vi "Taiko_SimpleDemo.vi"() -> ()   [LabVIEW 2017]
uses:
  _lib/PDLM/pdlm_lib_x86_x64_UIThread.llb/PDLM_LHData.ctl
  _lib/PDLM/pdlm_lib_x86_x64_UIThread.llb/PDLM_LHData_LaserType.ctl
  _lib/PDLM/pdlm_lib_x86_x64_UIThread.llb/PDLM_LHVersion.ctl
  _lib/PDLM/pdlm_lib_x86_x64_UIThread.llb/PDLM_SystemStatus.ctl
  _lib/PDLM/pdlm_lib_x86_x64_UIThread.llb/PDLM_LaserMode.ctl
  _lib/PDLM/pdlm_lib_x86_x64_UIThread.llb/PDLM_TaggedValueList.ctl
  _lib/PDLM/pdlm_lib_x86_x64_UIThread.llb/PDLM_TaggedValue.ctl
  _lib/PDLM/pdlm_lib_x86_x64_UIThread.llb/PDLM_Tag.ctl
  <vilib>/Utility/error.llb/Error Cluster From Error Code.vi
  _lib/PDLM/pdlm_lib_x86_x64_UIThread.llb/PDLM_DllPath_global.vi
  <vilib>/ErrorRing/Error Ring.xnode
panel:
  out "Errror":errorcluster
  in  "Exit":bool
  in  "Update":bool
  out "String":string
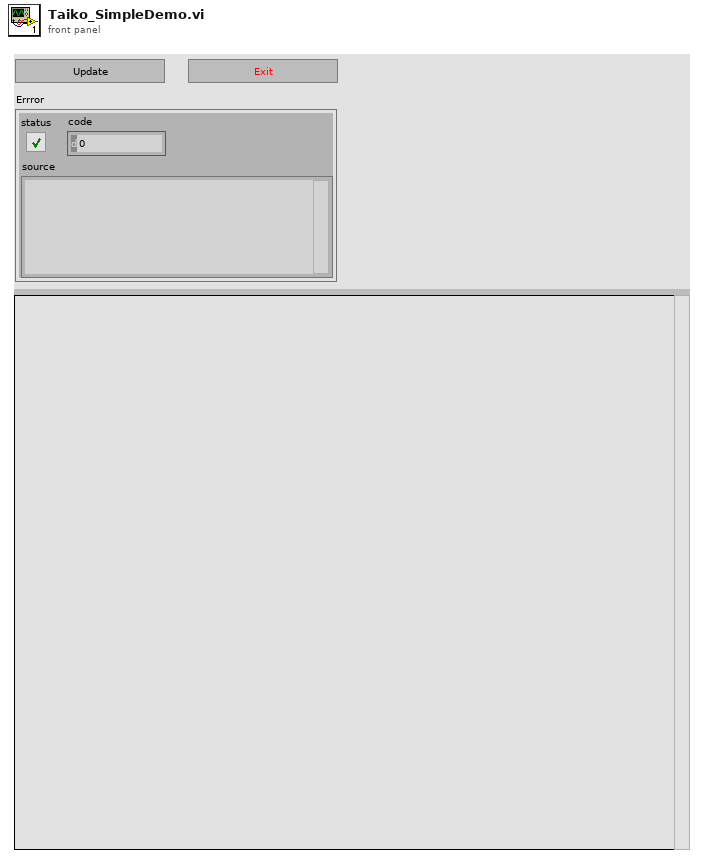
[diagram p1: front panel]
types:
  T1 = typedef "PDLM_LHData.ctl" = cluster{"SerNo":u32, "Features":u32, "FreqMin":u32, "FreqMax":u32, "CwPowerMax":u32, "PulsePowerMax":u32, "WavelengthNominal":u16, "CaseTempMax":u16, "Protection":bool, "LHTypeCtrlVoltage":u16, "LHMaxVoltage":u16, "CurrentTEP12V":u16, "LaserType":T2, "LHVersion":T3, "CalWarrentHours":u16}
  T2 = typedef "PDLM_LHData_LaserType.ctl" = u16
  T3 = typedef "PDLM_LHVersion.ctl" = cluster{"Major":u16, "Minor":u16}
  T4 = typedef "PDLM_LaserMode.ctl" = enum32{"CW", "PULSE", "BURST"}
  T5 = typedef "PDLM_TaggedValueList.ctl" = T6[]
  T6 = typedef "PDLM_TaggedValue.ctl" = cluster{"Tag":T7, "Value":u32}
  T7 = typedef "PDLM_Tag.ctl" = u32
  T8 = typedef "PDLM_SystemStatus.ctl" = u32
  T9 = typedef "PDLM_LHInfo.ctl" = cluster{"LType":string, "Date":string, "LClass":string}
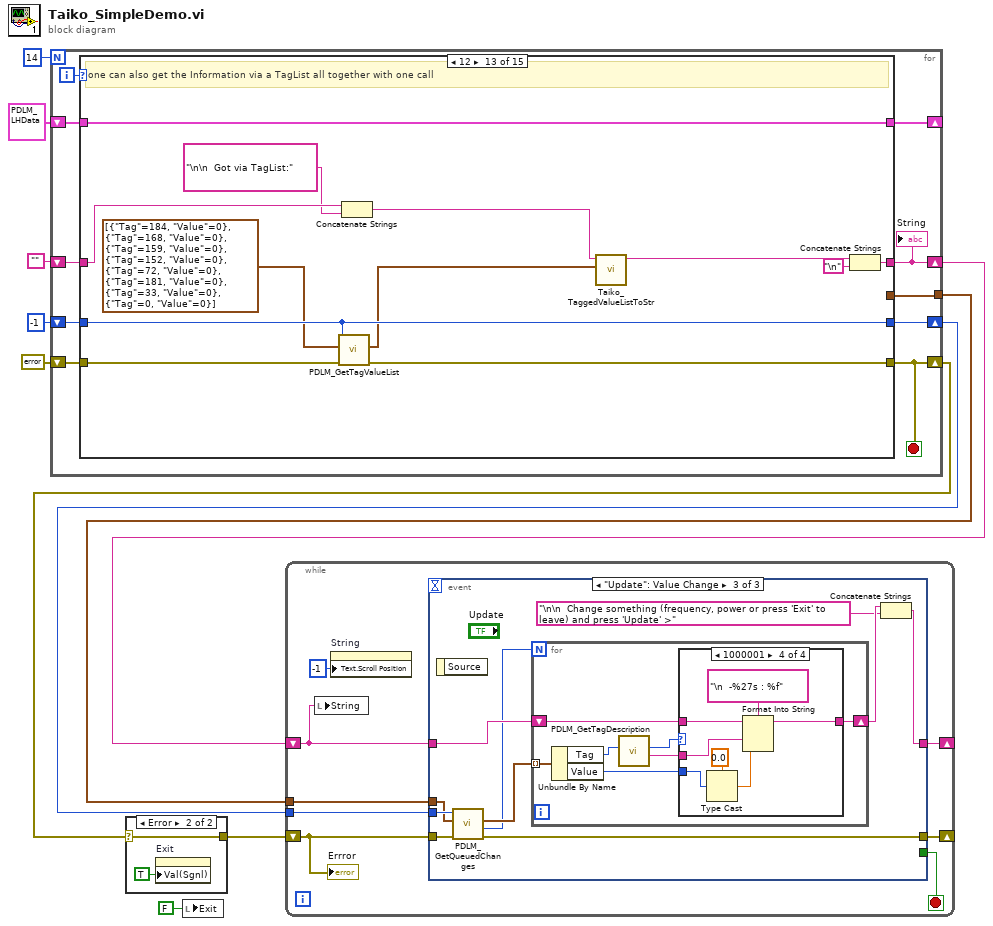
[diagram p0: block diagram]
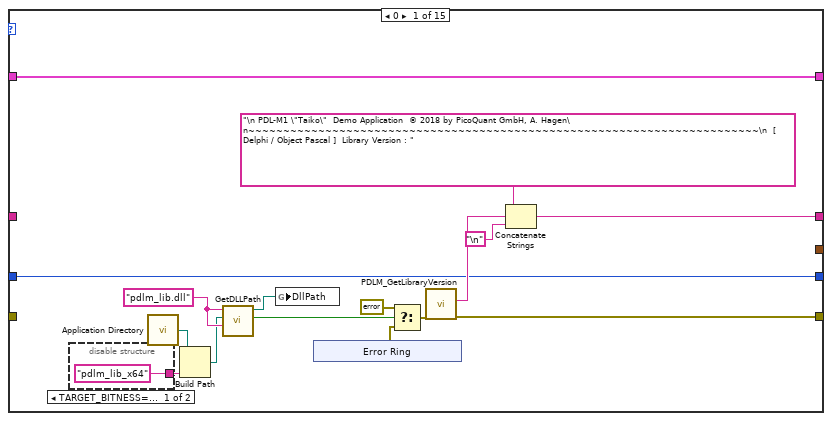
[diagram p3: hidden frame]
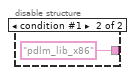
[diagram p4: hidden frame]
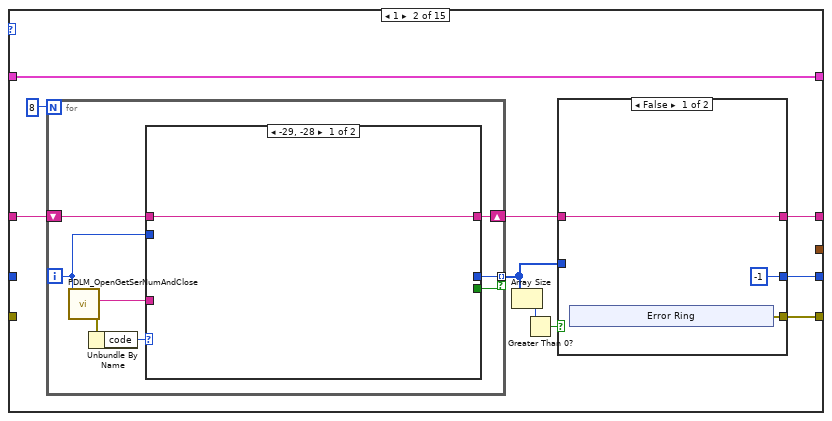
[diagram p5: hidden frame]
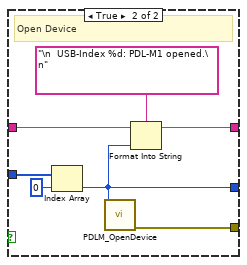
[diagram p6: hidden frame]
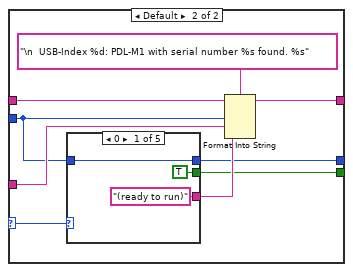
[diagram p7: hidden frame]
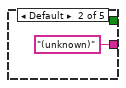
[diagram p8: hidden frame]
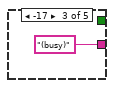
[diagram p9: hidden frame]
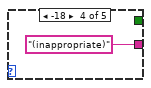
[diagram p10: hidden frame]
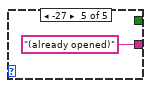
[diagram p11: hidden frame]
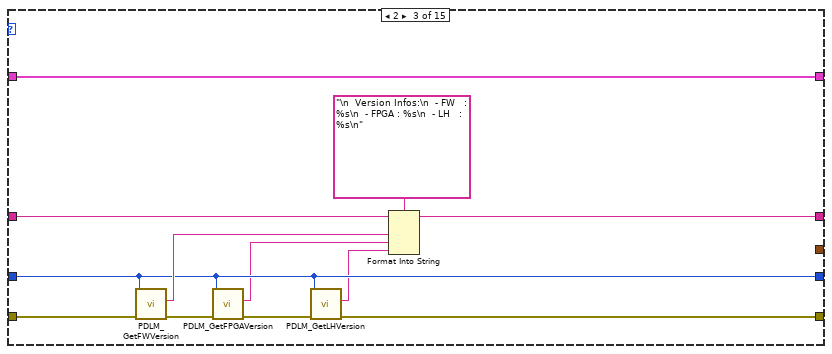
[diagram p12: hidden frame]
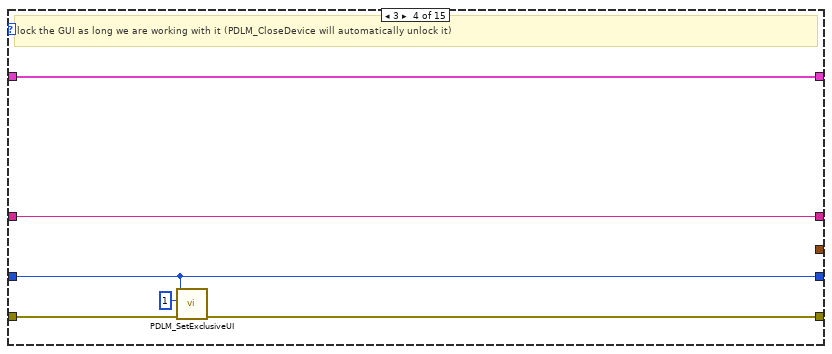
[diagram p13: hidden frame]
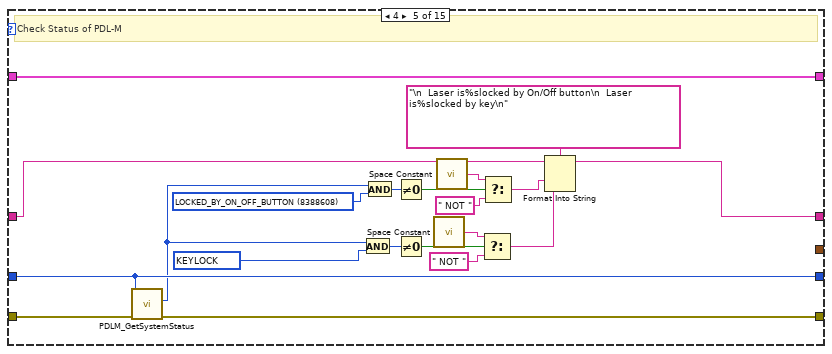
[diagram p14: hidden frame]
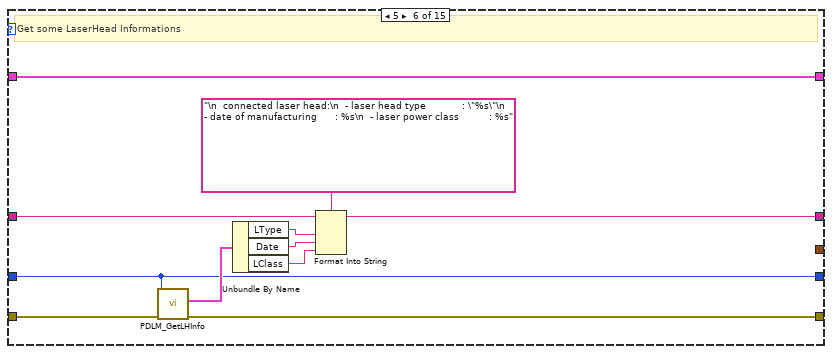
[diagram p15: hidden frame]
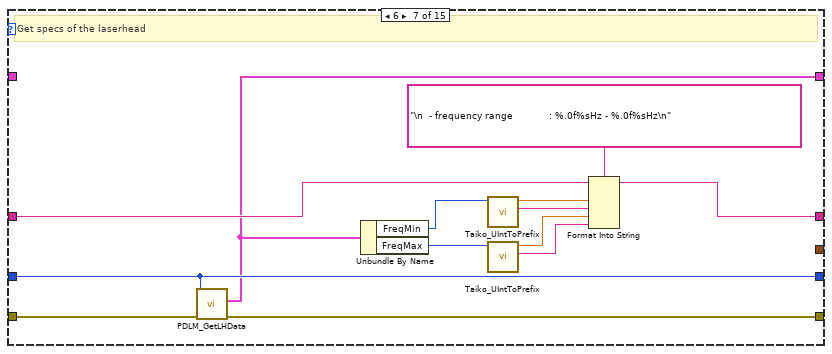
[diagram p16: hidden frame]
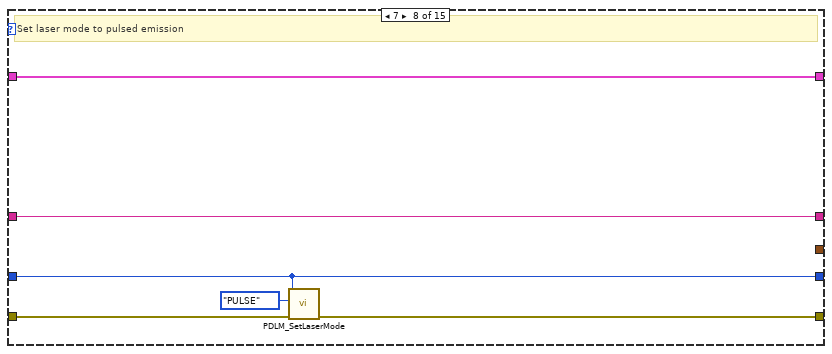
[diagram p17: hidden frame]
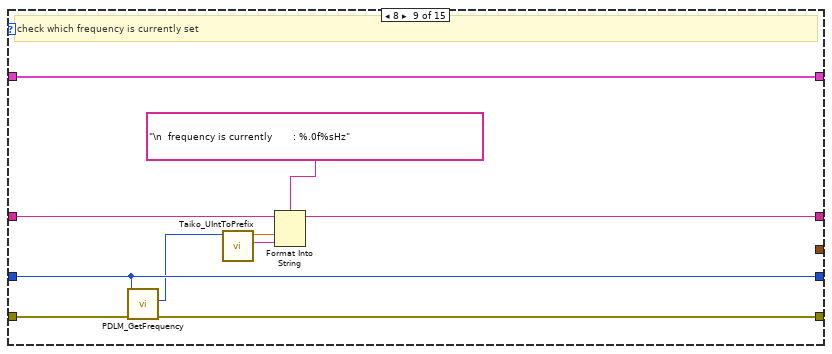
[diagram p18: hidden frame]
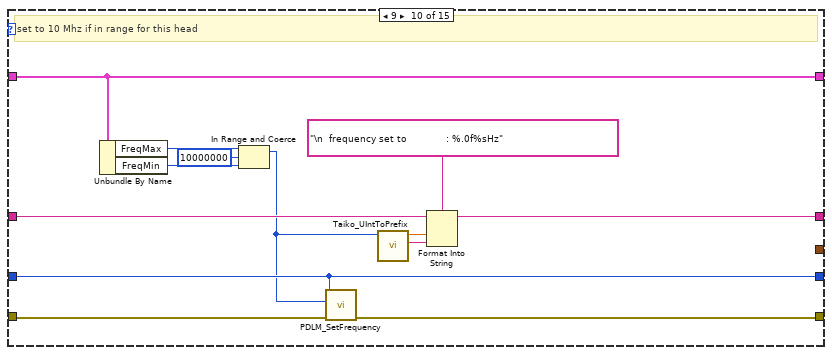
[diagram p19: hidden frame]
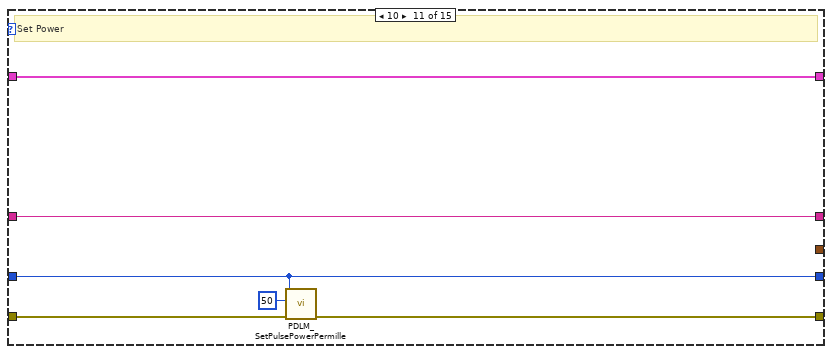
[diagram p20: hidden frame]
diagram:
  n1 = for {
    N: 14 -> [_]
    shift-right: [w15] -> w5
    shift-left: "" -> [w17]
    shift-right: [w16] -> w3
    shift-left: errorcluster {"status"=FALSE, "code"=0, "source"=""} ("error out") -> [w20]
    shift-right: [w18] -> w6
    shift-left: -1 -> [w19]
    shift-right: [w14] -> _
    shift-left: T1 {"SerNo"=0, "Features"=0, "FreqMin"=0, "FreqMax"=0, "CwPowerMax"=0, "PulsePowerMax"=0, "WavelengthNominal"=0, "CaseTempMax"=0, "Protection"=FALSE, "LHTypeCtrlVoltage"=0, "LHMaxVoltage"=0, "CurrentTEP12V"=0, "LaserType"=0, "LHVersion"={"Major"=0, "Minor"=0}, "CalWarrentHours"=0} ("Data") -> [w13]
    tunnel: [w12] -> w4
    i -> [w21]
    stop <- w16 stop-if-true
    n2 = case shown="12" w21 {
      tunnel: [w35 w47 w102 w108 w119 w134 w151 w158 w167 w177 w187 w196 w206 w218 w230] -> w15
      tunnel: [w34 w48 w96 w110 w131 w138 w154 w160 w170 w180 w189 w200 w211 w221 w232] -> w16
      tunnel: w20 -> [_ _ w106 w111 w132 w139 w155 w161 w171 w181 w190 w201 w212 w225 w232]
      tunnel: w19 -> [w33 _ w99 w109 w130 w137 w153 w159 w169 w179 w188 w195 w210 w220 w231]
      tunnel: [w33 w49 w99 w109 w130 w137 w153 w159 w169 w179 w188 w195 w210 w220 w231] -> w18
      tunnel: w17 -> [_ w53 w104 w108 w120 w135 w152 w158 w168 w178 w187 w197 w203 w219 w230]
      tunnel: [w31 w45 w95 w107 w117 w133 w150 w157 w166 w185 w186 w199 w213 w224 w229] -> w14
      tunnel: w13 -> [w31 w45 w95 w107 w117 w133 _ w157 w166 w185 w186 w199 w213 w224 w229]
      tunnel: [_ _ _ _ _ _ _ _ _ _ _ _ _ w214 _] -> w12
      frame 0 {
        w30 = "pdlm_lib.dll" ("DllName_64bit")
        n3 = disable-structure shown="TARGET_BITNESS==64, Default" {
          disable-tunnel: ["pdlm_lib_x64" "pdlm_lib_x86"] -> w28
          frame condition #0 (active) {
          }
          frame condition #1 {
          }
        }
        n4 = call <vilib>:"Application Directory.vi"() -> ("Application Directory"=w29:path)
        n5 = Build Path(base path=w29, name or relative path=w28) -> (appended path=w27:path)
        n6 = call "GetDLLPath.vi"("DllName_32bit"=w30, "PathToDLL"=w27, "DllName_64bit"=w30) -> ("file exists?"=w25:bool, "DLLPath"=w26:path)  [unwired: 7 in]
        n7 = global write "PDLM_DllPath_global.vi" "DllPath"(w26) -> ()
        n8 = xnode "Error Ring"() -> ("error out"=w22:errorcluster)
        n9 = Select(t=errorcluster {"status"=FALSE, "code"=0, "source"=""} ("error in (no error)"), s=w25, f=w22) -> (s? t:f=w23:errorcluster)
        n10 = call "PDLM_GetLibraryVersion.vi"("error in (no error)"=w23) -> ("error out"=w34:errorcluster, "Version"=w37:string)  [unwired: 8 in, 1 out]
        n11 = Concatenate Strings("\n PDL-M1 \"Taiko\"  Demo Application  © 2018 by PicoQuant GmbH, A. Hagen\n~~~~~~~~~~~~~~~~~~~~~~~~~~~~~~~~~~~~~~~~~~~~~~~~~~~~~~~~~~~~~~~~~~~~~~~~~\n  [ Delphi / Object Pascal ]  Library Version : ", w37, "\n") -> (w35:string)
      }
      frame 1 {
        n12 = for {
          N: 8 -> [_]
          tunnel: [w72] -> w50 mode=indexing if=w71
          shift-right: [w74] -> w46
          shift-left: w53 -> [w75]
          i -> [w73]
          n13 = call "PDLM_OpenGetSerNumAndClose.vi"("USBIdx"=w73) -> ("error out"=w76:errorcluster, "SerNo"=w77:string)  [unwired: 8 in, 1 out]
          n14 = Unbundle By Name(w76) -> ("code"=w70:i32)
          n15 = case shown="-29, -28" w70 {
            selector: w70 -> [_ w79]
            tunnel: w77 -> [_ w87]
            tunnel: w75 -> [w78 w84]
            tunnel: [w78 w83] -> w74
            tunnel: w73 -> [_ w82]
            tunnel: [_ w81] -> w72
            tunnel: [_ w80] -> w71
            frame -29, -28 {
            }
            frame Default {
              n16 = case shown="0" w79 {
                tunnel: ["(ready to run)" "(unknown)" "(busy)" "(inappropriate)" "(already opened)"] -> w86
                tunnel: w82 -> [w89 _ _ _ _]
                tunnel: [w89 _ _ _ _] -> w81
                tunnel: [TRUE _ _ _ _] -> w80
                frame 0 {
                }
                frame Default {
                }
                frame -17 {
                }
                frame -18 {
                }
                frame -27 {
                }
              }
              n17 = Format Into String(format string="\n  USB-Index %d: PDL-M1 with serial number %s found. %s", initial string=w84, w82, w87, w86) -> (resulting string=w83:string)  [unwired: 1 in, 1 out]
            }
          }
        }
        n18 = Array Size(array=w50) -> (size(s)=w52:i32)
        n19 = Greater Than 0?(x=w52) -> (x > 0?=w51:bool)
        n20 = case shown="False" w51 {
          tunnel: w50 -> [_ w69]
          tunnel: [-1 w64] -> w49
          tunnel: [w56 w67] -> w48
          tunnel: [w55 w65] -> w47
          tunnel: w46 -> [w55 w66]
          frame False {
            n21 = xnode "Error Ring"() -> ("error out"=w56:errorcluster)
          }
          frame True {
            # "Open Device"
            n22 = Index Array(array=w69, index=0) -> (element=w64:i32)
            n23 = call "PDLM_OpenDevice.vi"("USBIdx"=w64) -> ("error out"=w67:errorcluster)  [unwired: 8 in, 2 out]
            n24 = Format Into String(format string="\n  USB-Index %d: PDL-M1 opened.\n", initial string=w66, w64) -> (resulting string=w65:string)  [unwired: 1 in, 1 out]
          }
        }
      }
      frame 2 {
        n25 = call "PDLM_GetFWVersion.vi"("error in (no error)"=w106, "USBIdx"=w99) -> ("error out"=w101:errorcluster, "Version"=w105:string)  [unwired: 7 in, 1 out]
        n26 = call "PDLM_GetFPGAVersion.vi"("error in (no error)"=w101, "USBIdx"=w99) -> ("error out"=w100:errorcluster, "Version"=w98:string)  [unwired: 7 in, 1 out]
        n27 = call "PDLM_GetLHVersion.vi"("error in (no error)"=w100, "USBIdx"=w99) -> ("error out"=w96:errorcluster, "Version"=w97:string)  [unwired: 7 in, 1 out]
        n28 = Format Into String(format string="\n  Version Infos:\n  - FW   : %s\n  - FPGA : %s\n  - LH   : %s\n", initial string=w104, w105, w98, w97) -> (resulting string=w102:string)  [unwired: 1 in, 1 out]
      }
      frame 3 {
        # "lock the GUI as long we are working with it (PDLM_CloseDevice will automatically unlock it)"
        n29 = call "PDLM_SetExclusiveUI.vi"("error in (no error)"=w111, "mode"=u32 1, "USBIdx"=w109) -> ("error out"=w110:errorcluster)  [unwired: 7 in, 1 out]
      }
      frame 4 {
        w125 = T8 33554432 items=["INITIALIZING"=1, "DEVICE_UNCALIBRATED"=2, "COMMISSIONING_MODE"=4, "LASERHEAD_SAFETY_MODE"=8, "FW_UPDATE_RUNNING"=16, "DEVICE_DEFECT"=32, "DEVICE_INCOMPATIBLE"=64, "BUSY"=128, "EXCLUSIVE_SW_OP_GRANTED"=256, "PARAMETER_CHANGES_PENDING"=512, "LASERHEAD_CHANGED"=2048, "LASERHEAD_MISSING"=4096, "LASERHEAD_DEFECT"=8192, "LASERHEAD_UNKNOWN_TYPE"=16384, "LASERHEAD_DECALIBRATED"=32768, "LASERHEAD_DIODE_TEMP_TOO_LOW"=65536, "LASERHEAD_DIODE_TEMP_TOO_HIGH"=131072, "LASERHEAD_DIODE_OVERHEATING"=262144, "LASERHEAD_CASE_OVERHEATING"=524288, "LASERHEAD_FAN_RUNNING"=1048576, "LASERHEAD_INCOMPATIBLE"=2097152, "LOCKED_BY_EXPIRED_DEMO_MODE"=4194304, "LOCKED_BY_ON_OFF_BUTTON"=8388608, "SOFTLOCK"=16777216, "KEYLOCK"=33554432, "LOCKED_BY_SECURITY_POLICY"=67108864, "INTERLOCK"=134217728, "LASERHEAD_PULSE_POWER_INACCURATE"=268435456, "ERRORMSG_PENDING"=2147483648] ("SystemStatus")
        w124 = T8 8388608 items=["INITIALIZING"=1, "DEVICE_UNCALIBRATED"=2, "COMMISSIONING_MODE"=4, "LASERHEAD_SAFETY_MODE"=8, "FW_UPDATE_RUNNING"=16, "DEVICE_DEFECT"=32, "DEVICE_INCOMPATIBLE"=64, "BUSY"=128, "EXCLUSIVE_SW_OP_GRANTED"=256, "PARAMETER_CHANGES_PENDING"=512, "LASERHEAD_CHANGED"=2048, "LASERHEAD_MISSING"=4096, "LASERHEAD_DEFECT"=8192, "LASERHEAD_UNKNOWN_TYPE"=16384, "LASERHEAD_DECALIBRATED"=32768, "LASERHEAD_DIODE_TEMP_TOO_LOW"=65536, "LASERHEAD_DIODE_TEMP_TOO_HIGH"=131072, "LASERHEAD_DIODE_OVERHEATING"=262144, "LASERHEAD_CASE_OVERHEATING"=524288, "LASERHEAD_FAN_RUNNING"=1048576, "LASERHEAD_INCOMPATIBLE"=2097152, "LOCKED_BY_EXPIRED_DEMO_MODE"=4194304, "LOCKED_BY_ON_OFF_BUTTON"=8388608, "SOFTLOCK"=16777216, "KEYLOCK"=33554432, "LOCKED_BY_SECURITY_POLICY"=67108864, "INTERLOCK"=134217728, "LASERHEAD_PULSE_POWER_INACCURATE"=268435456, "ERRORMSG_PENDING"=2147483648] ("SystemStatus")
        # "Check Status of PDL-M"
        n30 = call "PDLM_GetSystemStatus.vi"("error in (no error)"=w132, "USBIdx"=w130) -> ("error out"=w131:errorcluster, "state"=w123:u32)  [unwired: 7 in, 1 out]
        n31 = And(x=w123, y=w125) -> (x .and. y?=w127:T8)
        n32 = And(x=w123, y=w124) -> (x .and. y?=w126:T8)
        n33 = Not Equal To 0?(x=w126) -> (x != 0?=w128:bool)
        n34 = Not Equal To 0?(x=w127) -> (x != 0?=w129:bool)
        n35 = call <vilib>:"Space Constant.vi"() -> ("String"=w116:string)
        n36 = call <vilib>:"Space Constant.vi"() -> ("String"=w114:string)
        n37 = Select(t=w116, s=w129, f=" NOT ") -> (s? t:f=w121:string)
        n38 = Select(t=w114, s=w128, f=" NOT ") -> (s? t:f=w122:string)
        n39 = Format Into String(format string="\n  Laser is%slocked by On/Off button\n  Laser is%slocked by key\n", initial string=w120, w122, w121) -> (resulting string=w119:string)  [unwired: 1 in, 1 out]
      }
      frame 5 {
        # "Get some LaserHead Informations"
        n40 = call "PDLM_GetLHInfo.vi"("error in (no error)"=w139, "USBIdx"=w137) -> ("error out"=w138:errorcluster, "LHInfo"=w140:T9)  [unwired: 7 in, 1 out]
        n41 = Unbundle By Name(w140) -> ("LType"=w141:string, "Date"=w142:string, "LClass"=w143:string)
        n42 = Format Into String(format string="\n  connected laser head:\n  - laser head type            : \"%s\"\n  - date of manufacturing      : %s\n  - laser power class          : %s", initial string=w135, w141, w142, w143) -> (resulting string=w134:string)  [unwired: 1 in, 1 out]
      }
      frame 6 {
        # "Get specs of the laserhead"
        n43 = call "PDLM_GetLHData.vi"("error in (no error)"=w155, "USBIdx"=w153) -> ("error out"=w154:errorcluster, "Data"=w150:T1)  [unwired: 7 in, 1 out]
        n44 = Unbundle By Name(w150) -> ("FreqMin"=w146:u32, "FreqMax"=w149:u32)
        n45 = call "Taiko_UIntToPrefix.vi"("UINT"=w146) -> ("PREFIX"=w144:string, "MANT"=w145:sgl)  [unwired: 9 in]
        n46 = call "Taiko_UIntToPrefix.vi"("UINT"=w149) -> ("PREFIX"=w147:string, "MANT"=w148:sgl)  [unwired: 9 in]
        n47 = Format Into String(format string="\n  - frequency range            : %.0f%sHz - %.0f%sHz\n", initial string=w152, w145, w144, w148, w147) -> (resulting string=w151:string)  [unwired: 1 in, 1 out]
      }
      frame 7 {
        # "Set laser mode to pulsed emission"
        n48 = call "PDLM_SetLaserMode.vi"("error in (no error)"=w161, "mode"=PDLM_LaserMode."PULSE", "USBIdx"=w159) -> ("error out"=w160:errorcluster)  [unwired: 7 in, 1 out]
      }
      frame 8 {
        # "check which frequency is currently set"
        n49 = call "PDLM_GetFrequency.vi"("error in (no error)"=w171, "USBIdx"=w169) -> ("error out"=w170:errorcluster, "freq"=w165:u32)  [unwired: 7 in, 1 out]
        n50 = call "Taiko_UIntToPrefix.vi"("UINT"=w165) -> ("PREFIX"=w163:string, "MANT"=w164:sgl)  [unwired: 9 in]
        n51 = Format Into String(format string="\n  frequency is currently       : %.0f%sHz", initial string=w168, w164, w163) -> (resulting string=w167:string)  [unwired: 1 in, 1 out]
      }
      frame 9 {
        # "set to 10 Mhz if in range for this head"
        n52 = Unbundle By Name(w185) -> ("FreqMax"=w184:u32, "FreqMin"=w183:u32)
        n53 = In Range and Coerce(upper limit=w184, x=u32 10000000 ("freq"), lower limit=w183) -> (coerced(x)=w175:u32)  [unwired: 1 out]
        n54 = call "PDLM_SetFrequency.vi"("error in (no error)"=w181, "freq"=w175, "USBIdx"=w179) -> ("error out"=w180:errorcluster)  [unwired: 7 in, 1 out]
        n55 = call "Taiko_UIntToPrefix.vi"("UINT"=w175) -> ("PREFIX"=w173:string, "MANT"=w174:sgl)  [unwired: 9 in]
        n56 = Format Into String(format string="\n  frequency set to             : %.0f%sHz", initial string=w178, w174, w173) -> (resulting string=w177:string)  [unwired: 1 in, 1 out]
      }
      frame 10 {
        # "Set Power"
        n57 = call "PDLM_SetPulsePowerPermille.vi"("error in (no error)"=w190, "permille"=u32 50, "USBIdx"=w188) -> ("error out"=w189:errorcluster)  [unwired: 7 in, 1 out]
      }
      frame 11 {
        # "read the resulting Power in mW"
        n58 = call "PDLM_GetPulsePower.vi"("error in (no error)"=w201, "USBIdx"=w195) -> ("error out"=w200:errorcluster, "Power"=w194:sgl)  [unwired: 7 in, 1 out]
        n59 = call "Taiko_SGLToPrefix.vi"("SGL"=w194) -> ("PREFIX"=w192:string, "MANT"=w193:sgl)  [unwired: 9 in]
        n60 = Format Into String(format string="\n  pulse power set to           : %.3f%sW", initial string=w197, w193, w192) -> (resulting string=w196:string)  [unwired: 1 in, 1 out]
      }
      frame 12 {
        # "one can also get the Information via a TagList all together with one call"
        n61 = call "PDLM_GetTagValueList.vi"("error in (no error)"=w212, "TaggedValueList"=T5 [{"Tag"=184, "Value"=0}, {"Tag"=168, "Value"=0}, {"Tag"=159, "Value"=0}, {"Tag"=152, "Value"=0}, {"Tag"=72, "Value"=0}, {"Tag"=181, "Value"=0}, {"Tag"=33, "Value"=0}, {"Tag"=0, "Value"=0}], "USBIdx"=w210) -> ("error out"=w211:errorcluster, "TaggedValueList out"=w208:T5)  [unwired: 6 in, 1 out]
        n62 = Concatenate Strings(w203, "\n\n  Got via TagList:" ("string")) -> (w204:string)
        n63 = call "Taiko_TaggedValueListToStr.vi"("TaggedValueList in"=w208, "String in"=w204) -> ("String out"=w207:string)  [unwired: 9 in]
        n64 = Concatenate Strings(w207, "\n") -> (w206:string)
      }
      frame 13 {
        # "Unlock the Device GUI and ask user to change something"
        n65 = call "PDLM_SetExclusiveUI.vi"("error in (no error)"=w225, "mode"=u32 0, "USBIdx"=w220) -> ("error out"=w223:errorcluster)  [unwired: 7 in, 1 out]
        n66 = flat-sequence {
          tunnel: w223 -> [w227]
          tunnel: [w227] -> w222
          frame #0 {
            n67 = Wait (ms)(milliseconds to wait=u32 100) -> ()  [unwired: 1 out]
          }
        }
        n68 = Initialize Array(cluster{"Tag":T7, "Value":u32} {"Tag"=0, "Value"=0} ("TaggedValue"), 50 ("dimension size")) -> (w214:cluster{"Tag":T7, "Value":u32}[])
        n69 = call "PDLM_GetQueuedChanges.vi"("error in (no error)"=w222, "TaggedValueList"=w214, "USBIdx"=w220) -> ("error out"=w221:errorcluster)  [unwired: 5 in, 3 out]
        n70 = Concatenate Strings(w219, "\n  Device GUI unlocked\n\n\n  Change something (frequency, power or press 'Exit' to leave) and press 'Update' >" ("string")) -> (w218:string)
      }
      frame Default {
      }
    }
    "String" <- w15
  }
  n71 = case shown="Error" w3 {
    selector: w3 -> [w233 w235]
    tunnel: [w233 w235] -> w2
    frame No Error {
    }
    frame Error {
      n72 = property on="Exit" class="Bool (strict)"("Val(Sgnl)"=TRUE ("Value (Signaling)")) -> ()  [unwired: 2 in, 2 out]
    }
  }
  n73 = local write "Exit"(FALSE ("Exit")) -> ()
  n74 = while {
    tunnel: w6 -> [w242]
    tunnel: w4 -> [w241]
    shift-right: [w240] -> _
    shift-left: w5 -> [w237]
    shift-right: [w239] -> _
    shift-left: w2 -> [w238]
    stop <- w243 stop-if-true
    n75 = local write "String"(w237) -> ()
    n76 = property on="String" class="Str"("Text.Scroll Position"=-1) -> ()  [unwired: 2 in, 2 out]
    n77 = event shown="[2] \"Update\": Value Change" {
      selector: _ -> [_ _ _]
      dyn-events: _ -> [_ _ _]
      timeout: _ -> [_ _ _]
      tunnel: [TRUE TRUE _] -> w243
      tunnel: w242 -> [w246 w250 w261]
      tunnel: w237 -> [w245 w248 w257]
      tunnel: w241 -> [_ _ w260]
      tunnel: [w245 w248 w252] -> w240
      tunnel: w238 -> [_ _ w259]
      tunnel: [w244 _ w258] -> w239
      event "Exit": Value Change {
        n78 = event-data() -> ()  [unwired: 1 in, 6 out]
        n79 = call "PDLM_CloseDevice.vi"("USBIdx"=w246) -> ("error out"=w244:errorcluster)  [unwired: 9 in, 1 out]
      }
      event Panel Close? {
        n80 = event-data() -> ()  [unwired: 1 in, 1 out]
        n81 = call "PDLM_CloseDevice.vi"("USBIdx"=w250) -> ()  [unwired: 9 in, 2 out]
        n82 = event-data("Discard?"=TRUE) -> ()  [unwired: 1 in, 1 out]
      }
      event "Update": Value Change {
        n83 = event-data() -> ()  [unwired: 1 in, 1 out]
        n84 = call "PDLM_GetQueuedChanges.vi"("error in (no error)"=w259, "TaggedValueList"=w260, "USBIdx"=w261) -> ("error out"=w258:errorcluster, "ListLen out"=w255:u32, "TaggedValueList out"=w256:T5)  [unwired: 5 in, 1 out]
        n85 = for {
          N: w255 -> [_]
          tunnel: w256 -> [w268] mode=indexing
          shift-right: [w264] -> w254
          shift-left: w257 -> [w263]
          n86 = Unbundle By Name(w268) -> ("Tag"=w267:T7, "Value"=w265:u32)
          n87 = call "PDLM_GetTagDescription.vi"("Tag"=w267) -> ("Name"=w266:string, "TypeCode"=w262:u32)  [unwired: 7 in, 2 out]
          n88 = case shown="1000001" w262 {
            tunnel: w266 -> [_ w274 w281 w288]
            tunnel: w265 -> [_ w272 w276 w283]
            tunnel: [w269 w271 w279 w286] -> w264
            tunnel: w263 -> [w269 w270 w278 w285]
            frame Default {
            }
            frame 1..69377 {
              n89 = Format Into String(format string="\n  -%27s : %d", initial string=w270, w274, w272) -> (resulting string=w271:string)  [unwired: 1 in, 1 out]
            }
            frame 1114113..16777215 {
              n90 = Type Cast(type=0, x=w276) -> (*(type *) &x=w275:i32)
              n91 = Format Into String(format string="\n  -%27s : %d", initial string=w278, w281, w275) -> (resulting string=w279:string)  [unwired: 1 in, 1 out]
            }
            frame 16777217 {
              n92 = Type Cast(type=sgl 0.0, x=w283) -> (*(type *) &x=w282:sgl)
              n93 = Format Into String(format string="\n  -%27s : %f", initial string=w285, w288, w282) -> (resulting string=w286:string)  [unwired: 1 in, 1 out]
            }
          }
        }
        n94 = Concatenate Strings(w254, "\n\n  Change something (frequency, power or press 'Exit' to leave) and press 'Update' >") -> (w252:string)
      }
    }
    "Errror" <- w238
  }
